vi "CameraServo.vi"(11 "Angle":i32) -> ()   [LabVIEW 2018]
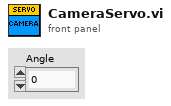
[diagram p1: front panel]
types:
  T1 = typedef "WPI_ServoDeviceRef.ctl" = cluster{"DeviceStatus":errorcluster, "PWM Channel":T2, "DeadBand":T3}
  T2 = typedef "FPGA_DIOPWMChannel.ctl" = enum8{"PWM 0", "PWM 1", "PWM 2", "PWM 3", "PWM 4", "PWM 5", "PWM 6", "PWM 7", "PWM 8", "PWM 9", "PWM MXP 0", "PWM MXP 1", "PWM MXP 2", "PWM MXP 3", "PWM MXP 4", "PWM MXP 5", "PWM MXP 6", "PWM MXP 7", "PWM MXP 8", "PWM MXP 9", "Invalid"}
  T3 = typedef "WPI_PWMDeadband.ctl" = cluster{"Name":string, "maxPositivePwm":i32, "minPositivePwm":i32, "centerPwm":i32, "maxNegativePwm":i32, "minNegativePwm":i32, "angularRange":u16}
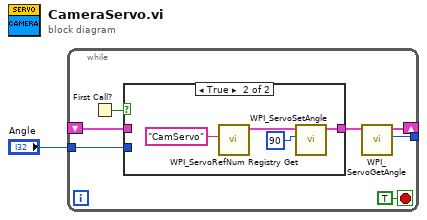
[diagram p0: block diagram]
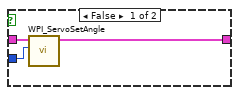
[diagram p2: hidden frame]
diagram:
  n1 = while {
    tunnel: "Angle" -> [w8]
    shift-right: [w3] -> _
    shift-left: _ -> [w7]
    tunnel: [w2] -> _
    stop <- TRUE stop-if-true
    n2 = First Call?() -> (First Call?: T/F=w5:bool)
    n3 = case shown="True" w5 {
      tunnel: w8 -> [w9 _]
      tunnel: [w11 w13] -> w4
      tunnel: w7 -> [w10 _]
      frame False {
        n4 = call <vilib>:"WPI_ServoSetAngle.vi"("Angle"=w9, "ServoDeviceRef"=w10) -> ("ServoDeviceRef"=w11:T1)  [unwired: 8 in, 1 out]
      }
      frame True {
        n5 = call <vilib>:"WPI_ServoRefNum Registry Get.vi"("refnum name"="CamServo") -> ("ServoDeviceRef"=w14:T1)  [unwired: 9 in, 1 out]
        n6 = call <vilib>:"WPI_ServoSetAngle.vi"("Angle"=90, "ServoDeviceRef"=w14) -> ("ServoDeviceRef"=w13:T1)  [unwired: 8 in, 1 out]
      }
    }
    n7 = call <vilib>:"WPI_ServoGetAngle.vi"("ServoDeviceRef"=w4) -> ("ServoDeviceRef"=w3:T1, "Angle"=w2:u16)  [unwired: 7 in, 1 out]
  }
